vi "UDP Core.vi"(6 "Timeouts":T4={"UDP Broadcast Link"=100, "Handle Failure Action"=10, "TCP Port Notification"=10}, 11 "Assert Message":T1) -> ()   [LabVIEW 2016, in "Assert API Components.lvlib" / "Log Assert Core.lvlib"]
uses:
  Log Assert Core.lvlib
  Timeouts.ctl
  Message Data.ctl
  Failure Actions.ctl
  VI References.ctl
  <vilib>/NI/STM/SubVIs/MetaDataElement.ctl
  <vilib>/NI/STM/UDP/UDP Read Options.ctl
  <vilib>/NI/STM/UDP/Write Message (UDP).vi
  <vilib>/NI/STM/UDP/Read Message (UDP).vi
  <vilib>/NI/STM/NI STM.lvlib
  Assert API Components.lvlib
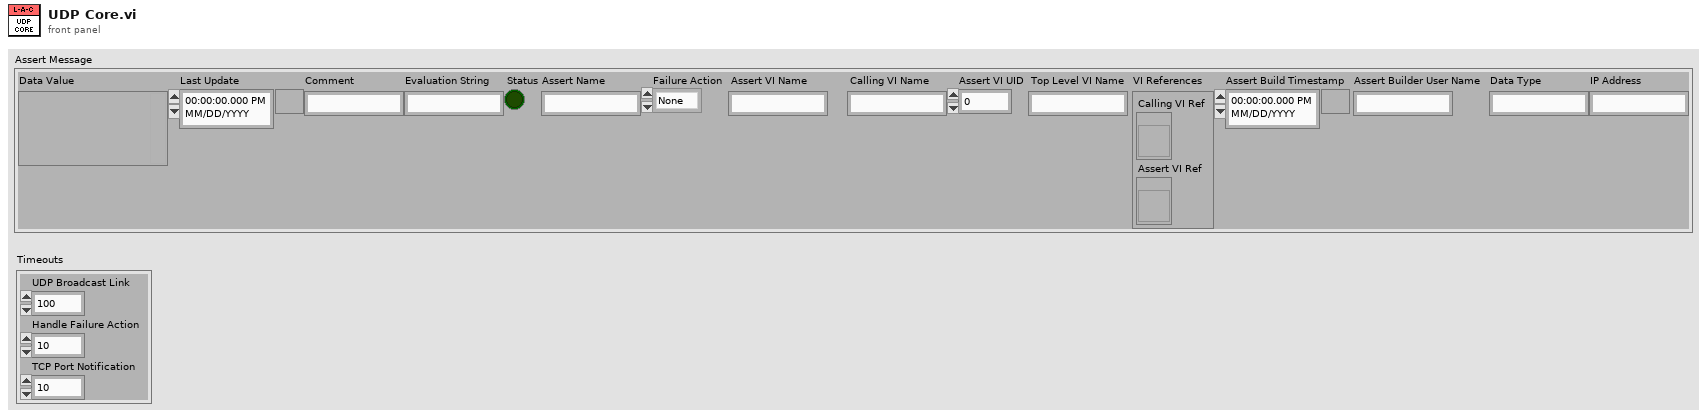
[diagram p1: front panel]
types:
  T1 = typedef "Assert API Components.lvlib/Message Data.ctl" = cluster{"Data Value":variant, "Last Update":timestamp, "Comment":string, "Evaluation String":string, "Status":bool, "Assert Name":string, "Failure Action":T2, "Assert VI Name":string, "Calling VI Name":string, "Assert VI UID":i32, "Top Level VI Name":string, "VI References":T3, "Assert Build Timestamp":timestamp, "Assert Builder User Name":string, "Data Type":string, "IP Address":string}
  T2 = typedef "Assert API Components.lvlib/Failure Actions.ctl" = enum16{"None", "Log To File", "Pause Execution", "Abort Execution"}
  T3 = typedef "Assert API Components.lvlib/VI References.ctl" = cluster{"Calling VI Ref":refnum<vi>, "Assert VI Ref":refnum<vi>}
  T4 = typedef "Assert API Components.lvlib/Timeouts.ctl" = cluster{"UDP Broadcast Link":i32, "Handle Failure Action":i32, "TCP Port Notification":i32}
  T5 = typedef "NI STM.lvlib/UDP Read Options.ctl" = cluster{"ignore timeout error":bool, "timeout ms (1000)":i32, "max size (548)":i32}
  T6 = typedef "NI STM.lvlib/MetaDataElement.ctl" = string
  T7 = typedef "NI STM.lvlib/UDP Connection Info.ctl" = cluster{"connection ID":refnum<k16>, "meta data":T6[]}
  T8 = typedef "NI STM.lvlib/UDP Data Info.ctl" = cluster{"address":u32, "port":u16, "bytes read":i32}
  T9 = typedef "NI STM.lvlib/TCP Connection Info.ctl" = cluster{"connection ID":refnum<k5>, "meta data":T6[]}
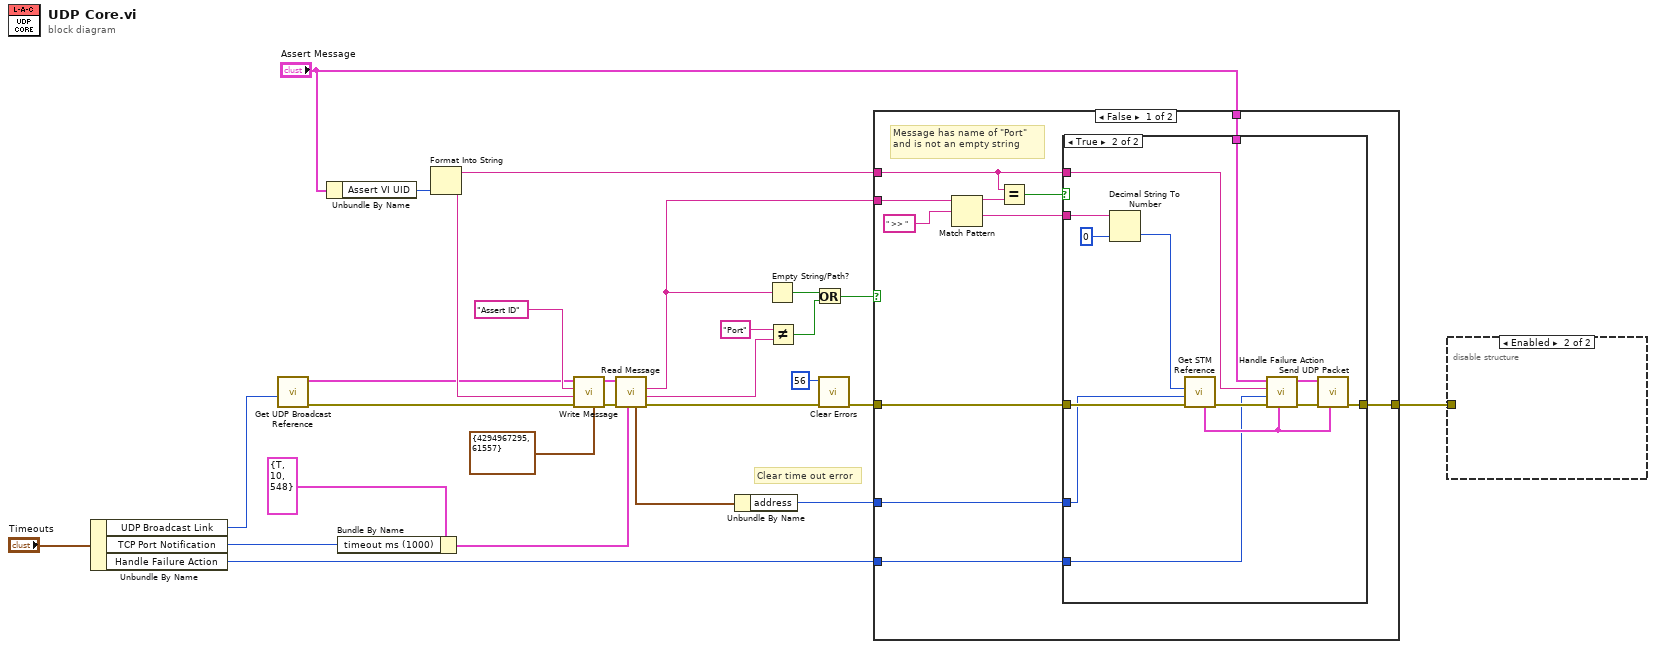
[diagram p0: block diagram]
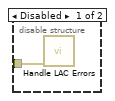
[diagram p4: hidden frame]
diagram:
  # "Clear time out error"
  n1 = Unbundle By Name("Timeouts") -> ("UDP Broadcast Link"=w6:i32, "TCP Port Notification"=w3:i32, "Handle Failure Action"=w5:i32)
  n2 = call "Get UDP Broadcast Reference.vi"("UDP Broadcast Link Timeout"=w6) -> ("error out"=w26:errorcluster, "Connection info out"=w14:T7)  [unwired: 9 in]
  n3 = Unbundle By Name("Assert Message") -> ("Assert VI UID"=w1:i32)
  n4 = Bundle By Name(cluster=T5 {"ignore timeout error"=TRUE, "timeout ms (1000)"=10, "max size (548)"=548} ("options 2"), "timeout ms (1000)"=w3) -> (w4:T5)
  n5 = Format Into String(w1) -> (resulting string=w19:string)  [unwired: 3 in, 1 out]
  n6 = call-poly <vilib>:"Write Message.vi"("address"=cluster{"address":u32, "port":u16} {"address"=4294967295, "port"=61557}, "error in"=w26, "data"=w19, "name"="Assert ID", "connection info in"=w14) -> ("error out"=w9:errorcluster, "connection info out"=w8:T7)  [unwired: 5 in]
  n7 = call-poly <vilib>:"Read Message.vi"("options"=w4, "error in"=w9, "connection info in"=w8) -> ("error out"=w24:errorcluster, "name"=w17:T6, "data string"=w13:string, "data info"=w12:T8)  [unwired: 3 in, 2 out]
  n8 = Unbundle By Name(w12) -> ("address"=w11:u32)
  n9 = Empty String/Path?(string/path=w13) -> (empty?=w16:bool)
  n10 = Not Equal?(x=T6 "Port" ("name 2"), y=w17) -> (x != y?=w15:bool)
  n11 = Or(x=w16, y=w15) -> (x .or. y?=w10:bool)
  n12 = call <vilib>:"Clear Errors.vi"("error in (no error)"=w24, "specific error code to clear (0: all)"=56) -> ("error out"=w20:errorcluster)  [unwired: 4 in, 1 out]
  n13 = case shown="False" w10 {
    tunnel: "Assert Message" -> [w38 _]
    tunnel: [w37 w53] -> w27
    tunnel: w20 -> [w35 w53]
    tunnel: w19 -> [w32 _]
    tunnel: w13 -> [w34 _]
    tunnel: w11 -> [w30 _]
    tunnel: w5 -> [w28 _]
    frame False {
      # "Message has name of \"Port\" and is not an empty string"
      n14 = Match Pattern(string=w34, regular expression=" >> ") -> (before substring=w33:string, after substring=w31:string)  [unwired: 1 in, 2 out]
      n15 = Equal?(x=w32, y=w33) -> (x = y?=w29:bool)
      n16 = case shown="True" w29 {
        tunnel: w38 -> [_ w52]
        tunnel: [w39 w51] -> w37
        tunnel: w35 -> [w39 w48]
        tunnel: w32 -> [_ w41]
        tunnel: w31 -> [_ w47]
        tunnel: w30 -> [_ w42]
        tunnel: w28 -> [_ w40]
        frame False {
          # "Not a message intended for this assert vi"
        }
        frame True {
          n17 = Decimal String To Number(string=w47, default (0L)=u16 0 ("default (0 I32)")) -> (number=w43:u16)  [unwired: 1 in, 1 out]
          n18 = call "Get STM Reference.vi"("error in (no error)"=w48, "IP Address"=w42, "Port"=w43) -> ("error out"=w45:errorcluster, "connection info out"=w44:T9)  [unwired: 7 in]
          n19 = call "Handle Failure Action.vi"("connection info in"=w44, "error in (no error)"=w45, "Handle Failure Action Timeout (ms)"=w40, "Assert UID"=w41, "Assert Message in"=w52) -> ("error out"=w50:errorcluster, "Assert Message out"=w49:T1)  [unwired: 5 in]
          n20 = call "Send UDP Packet.vi"("connection info in"=w44, "error in (no error)"=w50, "Assert Message in"=w49) -> ("error out"=w51:errorcluster)  [unwired: 8 in]
        }
      }
    }
    frame True {
      # "Not a valid message"
    }
  }
  n21 = disable-structure shown="Enabled" {
    disable-tunnel: w27 -> [w54 _]
    frame Disabled {
      n22 = call "Handle LAC Errors.vi"("error in (no error)"=w54) -> ()  [unwired: 11 in]
    }
    frame Enabled {
    }
  }
